vi "Configure Range Table (Spurious Emissions - Sweep And Limit).vi"(0 "VISA resource name":refnum<visa-resource-name>, 1 "Absolute Start Limit List":dbl[](array[numeric])=[-50.0, -50.0] format="%#.6g", 2 "Auto Points Mode List":bool[](array[boolean])=[FALSE, FALSE], 5 "Auto Sweep Time Mode List":bool[](array[boolean])=[TRUE, TRUE], 7 "Manual Sweep Time List":dbl[](array[numeric])=[0.001, 0.001], 9 "Auto Absolute Stop Limit  List":bool[](array[boolean])=[TRUE, TRUE], 11 "error in (no error)":errorcluster, 12 "Manual Absolute Stop Limit List":dbl[](array[numeric])=[-50.0, -50.0] format="%#.6g", 13 "Points Per Sweep List":i32[](array[numeric])=[601, 601]) -> (4 "VISA resource name out":refnum<visa-resource-name>, 15 "error out":errorcluster)   [LabVIEW 2014, in "Agilent MXA Series.lvlib"]
doc: "Configures the Sweep and Limit settings under Range Table for Spurious Emissions measurement type."
uses:
  Agilent MXA Series.lvlib
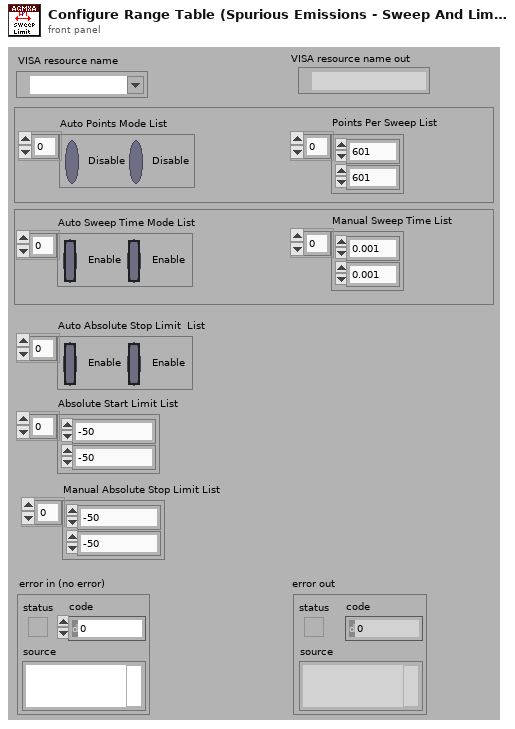
[diagram p1: front panel]
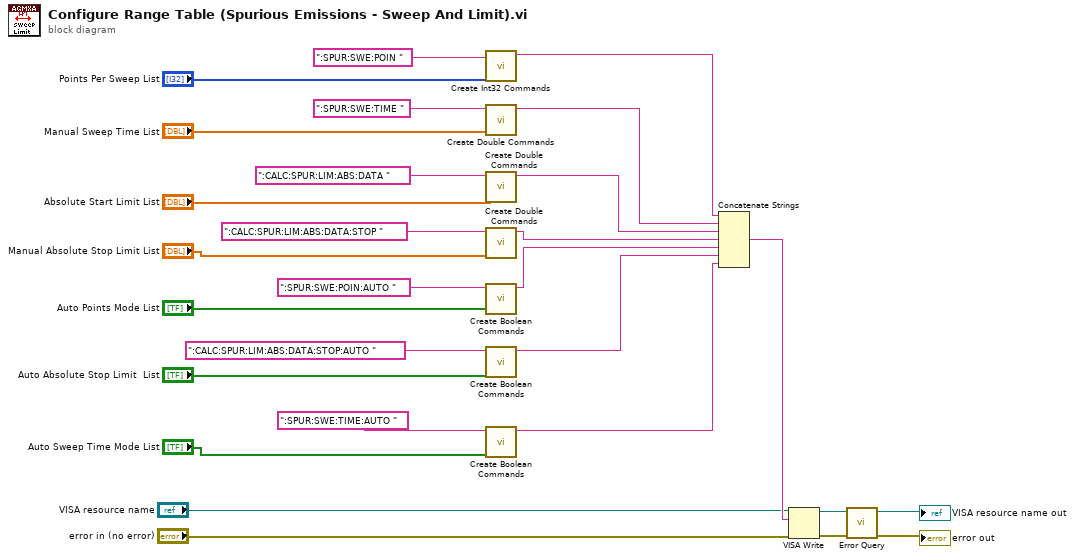
[diagram p0: block diagram]
diagram:
  n1 = call "Create Int32 Commands.vi"("Int Values"="Points Per Sweep List", "Commands"=":SPUR:SWE:POIN ") -> ("Result"=w1:string)  [unwired: 9 in]
  n2 = call "Create Double Commands.vi"("Double Values"="Manual Sweep Time List", "Commands"=":SPUR:SWE:TIME ") -> ("Result"=w16:string)  [unwired: 9 in]
  n3 = call "Create Double Commands.vi"("Double Values"="Absolute Start Limit List", "Commands"=":CALC:SPUR:LIM:ABS:DATA ") -> ("Result"=w15:string)  [unwired: 9 in]
  n4 = call "Create Double Commands.vi"("Double Values"="Manual Absolute Stop Limit List", "Commands"=":CALC:SPUR:LIM:ABS:DATA:STOP ") -> ("Result"=w14:string)  [unwired: 9 in]
  n5 = call "Create Boolean Commands.vi"("Boolean States"="Auto Points Mode List", "Command"=":SPUR:SWE:POIN:AUTO ") -> ("Result String"=w13:string)  [unwired: 9 in]
  n6 = call "Create Boolean Commands.vi"("Boolean States"="Auto Absolute Stop Limit  List", "Command"=":CALC:SPUR:LIM:ABS:DATA:STOP:AUTO ") -> ("Result String"=w12:string)  [unwired: 9 in]
  n7 = call "Create Boolean Commands.vi"("Boolean States"="Auto Sweep Time Mode List", "Command"=":SPUR:SWE:TIME:AUTO ") -> ("Result String"=w11:string)  [unwired: 9 in]
  n8 = Concatenate Strings(w1, w16, w15, w14, w13, w12, w11) -> (w10:string)
  n9 = VISA Write(VISA resource name="VISA resource name", write buffer=w10, error in (no error)="error in (no error)") -> (VISA resource name out=w6:refnum<visa-resource-name>, error out=w7:errorcluster)  [unwired: 1 out]
  n10 = call "Error Query.vi"("error in (no error)"=w7, "VISA resource name"=w6) -> ("error out"=→"error out":errorcluster, "VISA resource name out"=→"VISA resource name out":refnum<visa-resource-name>)  [unwired: 6 in, 2 out]
